vi "read_Fe.vi"() -> (0 "Fe H2 Dilute":bool, 1 "Actual Fe Flow Rate 3 (Vent)":dbl, 2 "Actual Fe Flow Rate2 (Bubbler)":dbl, 3 "Actual Fe Flow Rate1  (Out)":dbl, 4 "Fe Remote":bool, 5 "Fe Run":bool, 6 "Fe Bubbler":bool, 7 "Fe Active":bool)   [LabVIEW 2011]
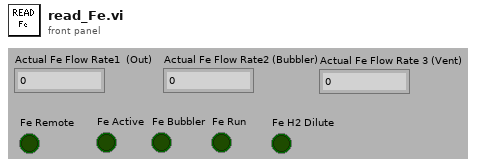
[diagram p1: front panel]
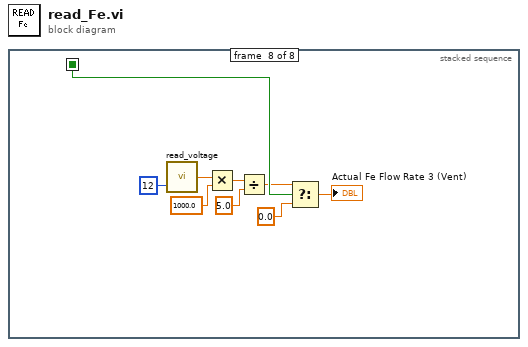
[diagram p0: block diagram]
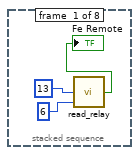
[diagram p2: hidden frame]
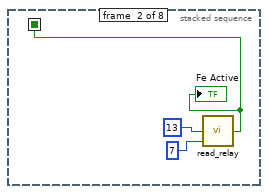
[diagram p3: hidden frame]
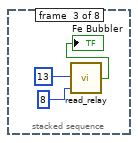
[diagram p4: hidden frame]
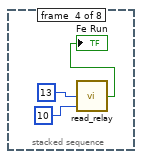
[diagram p5: hidden frame]
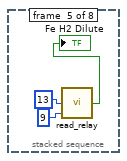
[diagram p6: hidden frame]
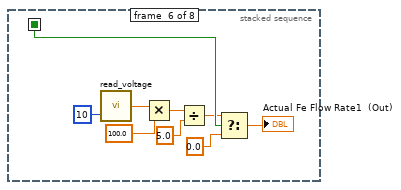
[diagram p7: hidden frame]
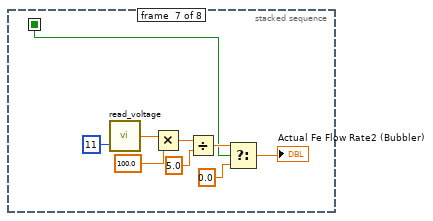
[diagram p8: hidden frame]
diagram:
  n1 = stacked-sequence {
    seq-local: [_ w4 _ _ _ _ _ _] -> [_ _ _ _ _ w19 w27 w37]
    frame #0 {
      n2 = call "read_relay.vi"("Relay"=6, "Slot"=13) -> ("Relay Status"=→"Fe Remote":bool)  [unwired: 1 out]
    }
    frame #1 {
      n3 = call "read_relay.vi"("Relay"=7, "Slot"=13) -> ("Relay Status"=w4:bool)  [unwired: 1 out]
      "Fe Active" <- w4
    }
    frame #2 {
      n4 = call "read_relay.vi"("Relay"=8, "Slot"=13) -> ("Relay Status"=→"Fe Bubbler":bool)  [unwired: 1 out]
    }
    frame #3 {
      n5 = call "read_relay.vi"("Relay"=10, "Slot"=13) -> ("Relay Status"=→"Fe Run":bool)  [unwired: 1 out]
    }
    frame #4 {
      n6 = call "read_relay.vi"("Relay"=9, "Slot"=13) -> ("Relay Status"=→"Fe H2 Dilute":bool)  [unwired: 1 out]
    }
    frame #5 {
      n7 = call "read_voltage.vi"("Channel"=10) -> ("Voltage"=w23:dbl)  [unwired: 1 in]
      n8 = Multiply(x=w23, y=100.0) -> (x*y=w21:dbl)
      n9 = Divide(x=w21, y=5.0) -> (x/y=w18:dbl)
      n10 = Select(t=w18, s=w19, f=0.0) -> (s? t:f=→"Actual Fe Flow Rate1  (Out)":dbl)
    }
    frame #6 {
      n11 = call "read_voltage.vi"("Channel"=11) -> ("Voltage"=w32:dbl)  [unwired: 1 in]
      n12 = Multiply(x=w32, y=100.0) -> (x*y=w30:dbl)
      n13 = Divide(x=w30, y=5.0) -> (x/y=w28:dbl)
      n14 = Select(t=w28, s=w27, f=0.0) -> (s? t:f=→"Actual Fe Flow Rate2 (Bubbler)":dbl)
    }
    frame #7 {
      n15 = call "read_voltage.vi"("Channel"=12) -> ("Voltage"=w41:dbl)  [unwired: 1 in]
      n16 = Multiply(x=w41, y=1000.0) -> (x*y=w39:dbl)
      n17 = Divide(x=w39, y=5.0) -> (x/y=w36:dbl)
      n18 = Select(t=w36, s=w37, f=0.0) -> (s? t:f=→"Actual Fe Flow Rate 3 (Vent)":dbl)
    }
  }
